vi "Async_Dialog.vi"(8 "error in (no error)":errorcluster, 10 "Dialog Text In":string, 11 "MHL_Data":T1) -> (0 "error out":errorcluster, 3 "MHL_Data 2":T1)   [LabVIEW 2019, in "MHL.lvlib"]
uses:
  MHL.lvlib
  typedef/MHL_Data.ctl
  Alarm_Panel/Channel_Temperature_Threshold.ctl
panel:
  in  "OK":bool
  out "Dialog Text":string
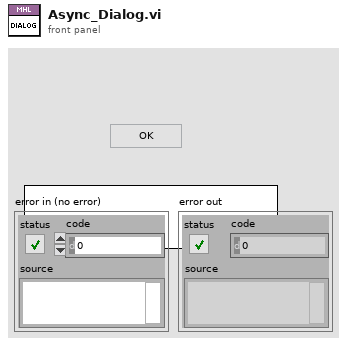
[diagram p1: front panel]
types:
  T1 = typedef "MHL.lvlib/MHL_Data.ctl" = cluster{"Ctrl_Refs":cluster{"Quit":refnum<vi>, "Motor_Switch":refnum<vi>, "Status":refnum<vi>, "Alarm_Panel":refnum<vi>, "Bearing Temp Chart":refnum<vi>, "Motor Temp Chart":refnum<vi>, "TabCtl":refnum<vi>, "Bearing Temp Clust":refnum<vi>}, "Main_Ref":refnum<vi>}
  T2 = enum8{"Enabled", "Disabled", "Disabled and Grayed Out"}
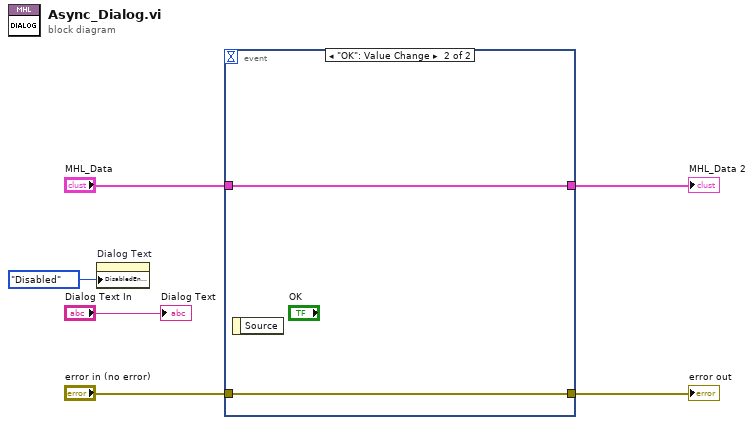
[diagram p0: block diagram]
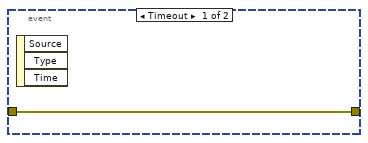
[diagram p2: hidden frame]
diagram:
  n1 = property on="Dialog Text" class="Str"("DisabledEnum"=T2."Disabled" ("Disabled")) -> ()  [unwired: 2 in, 2 out]
  n2 = event shown="[1] \"OK\": Value Change" {
    selector: _ -> [_ _]
    dyn-events: _ -> [_ _]
    timeout: _ -> [_ _]
    tunnel: "error in (no error)" -> [w7 w9]
    tunnel: [w7 w9] -> w4
    tunnel: "MHL_Data" -> [_ w8]
    tunnel: [_ w8] -> w1
    event Timeout {
      n3 = event-data() -> ()  [unwired: 1 in, 3 out]
    }
    event "OK": Value Change {
      n4 = event-data() -> ()  [unwired: 1 in, 1 out]
    }
  }
  "MHL_Data 2" <- w1
  "error out" <- w4
  "Dialog Text" <- "Dialog Text In"
